vi "Build Hierarchy Generator.vi"(0 "Build Analyzer in":refnum<class "Build Analyzer.lvclass">, 11 "error in (no error)":errorcluster) -> (4 "dup Build Analyzer":refnum<class "Build Analyzer.lvclass">, 6 "Top Down Working Set":refnum<data-value>, 15 "error out":errorcluster)   [LabVIEW 2017, in "CL_G3_VIComponentBuilder.lvlib" / "Build Analyzer.lvclass"]
doc: "Generates the a hierarchy of exports where each node in the hierarchy has as its child nodes the exports that it DEPENDS ON."
uses:
  Build Analyzer.lvclass
  <userlib>/_Cirrus Logic/LabVIEW Container/Source/Container/Container.lvclass
  Build Analyzer.lvclass/Build Analyzer.ctl
  <userlib>/_Cirrus Logic/LabVIEW Container/Source/Container/Get All Children.vi
  <userlib>/_Cirrus Logic/LabVIEW Container/Source/Container/GetAttribute_String.vi
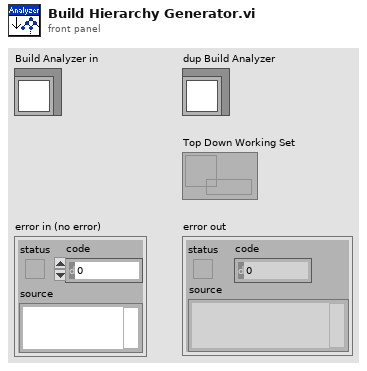
[diagram p1: front panel]
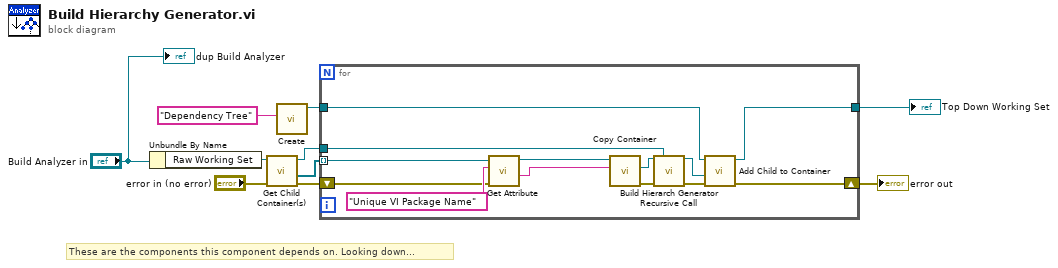
[diagram p0: block diagram]
diagram:
  # "These are the components this component depends on. Looking down..."
  n1 = Unbundle By Name("Build Analyzer in") -> ("Raw Working Set"=w7:refnum<data-value>)
  n2 = call-poly <userlib>:"Get Child Container(s).vi"("error in (no error)"="error in (no error)", "Container"=w7) -> ("error out"=w4:errorcluster, "Child Containers"=w10:refnum<data-value>[], "dup Container"=w1:refnum<data-value>)  [unwired: 6 in, 1 out]
  n3 = call <userlib>:"Create.vi"("Container Name"="Dependency Tree" ("New Container Name")) -> ("Container"=w9:refnum<data-value>)  [unwired: 9 in, 1 out]
  n4 = for {
    tunnel: w9 -> [w23]
    tunnel: w1 -> [w12]
    tunnel: [w21] -> w6
    tunnel: w10 -> [w20] mode=indexing
    shift-right: [w13] -> w3
    shift-left: w4 -> [w16]
    n5 = call-poly <userlib>:"Get Attribute.vi"("error in (no error)"=w16, "Attribute Name"="Unique VI Package Name", "Container Reference"=w20) -> ("String"=w17:string, "Container Reference out"=w11:refnum<data-value>)  [unwired: 5 in, 2 out]
    n6 = call <userlib>:"Copy Container.vi"("New Container Name"=w17, "Container"=w11) -> ("error out"=w15:errorcluster, "New Container"=w18:refnum<data-value>)  [unwired: 7 in, 1 out]
    n7 = call "Build Hierarch Generator Recursive Call.vi"("Node"=w18, "Working Set"=w12, "error in (no error)"=w15) -> ("Data Value Reference out"=w22:refnum<data-value>, "error out"=w14:errorcluster)  [unwired: 11 in]
    n8 = call <userlib>:"Add Child to Container.vi"("error in (no error)"=w14, "Child Container"=w22, "Container"=w23) -> ("error out"=w13:errorcluster, "dup Container"=w21:refnum<data-value>)  [unwired: 6 in, 1 out]
  }
  "error out" <- w3
  "Top Down Working Set" <- w6
  "dup Build Analyzer" <- "Build Analyzer in"
